vi "FormatTest.vi"(8 "entrée d'erreur (pas d'erreur)":errorcluster, 11 "read buffer en entrée":string) -> (0 "sortie d'erreur":errorcluster, 2 "result string":string)   [LabVIEW 2020]
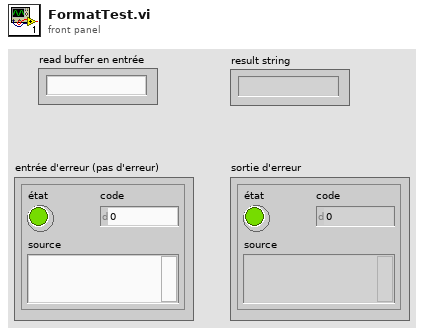
[diagram p1: front panel]
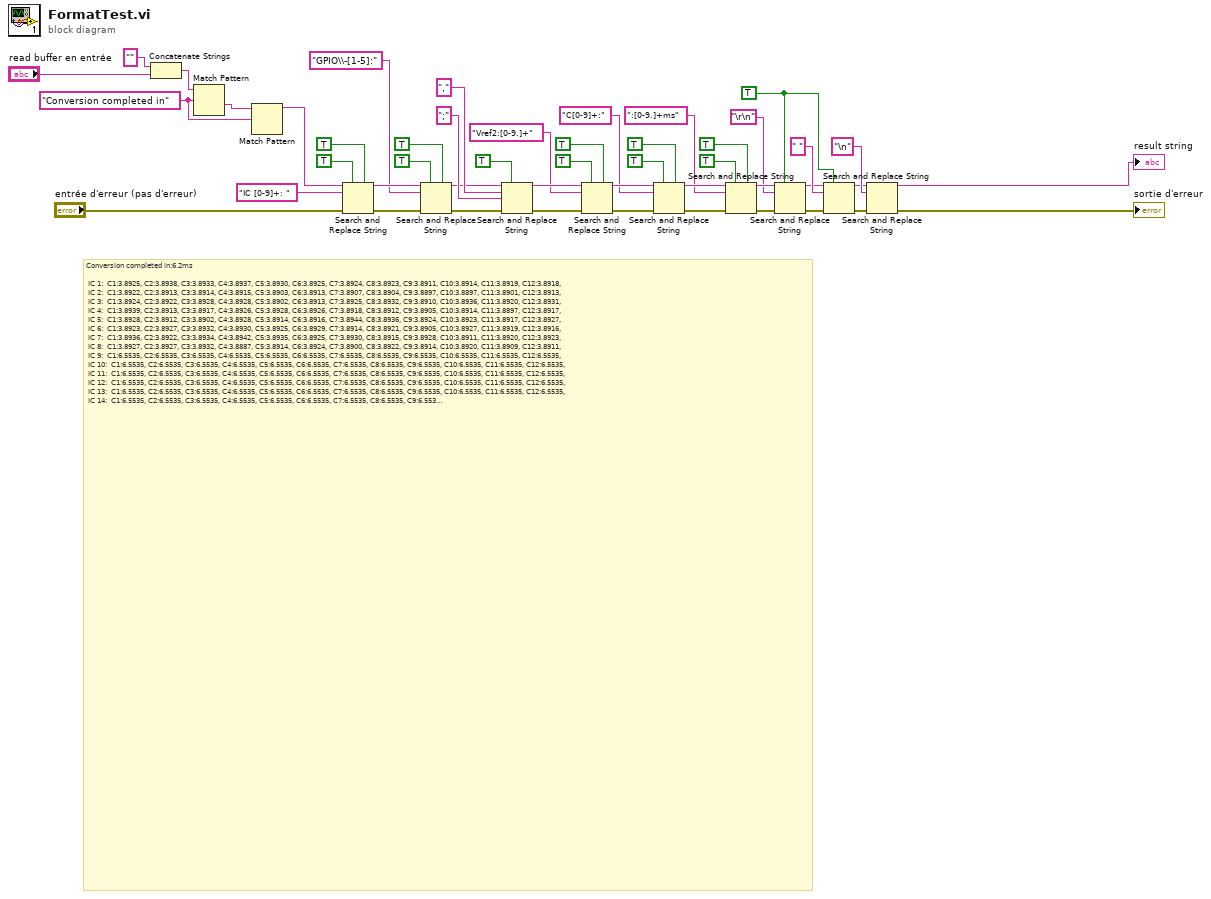
[diagram p0: block diagram]
diagram:
  w35 = "Conversion completed in" ("expression régulière")
  w24 = TRUE ("tout remplacer ? (F)")
  # "Conversion completed in:6.2ms \n\n IC 1:  C1:3.8925, C2:3.8938, C3:3.8933, C4:3.8937, C5:3.8930, C6:3.8925, C7:3.8924, C8:3.8923, C9:3.8911, C10:3.8914, C11:3.8919, C12:3.8918,\n IC 2:  C1:3.8922, C2:3.8913, C3:3.8914, C4:3.8915, C5:3.8903, C6:3.8913, C7:3.8907, C8:3.8904, C9:3.8897, C10:3.8897, C11:3.8901, C12:3.8913,\n IC 3:  C1:3.8924, C2:3.8922, C3:3.8928, C4:3.8928, C5:3.8902, C6:3.8913, C7:3.8925, C8:3.8932, C9:3.8910, C10:3.8936, C11:3.8920, C12:3.8931,\n IC 4:  C1:3.8939, C2:3.8913, C3:3.8917, C4:3.8926, C5:3.8928, C6:3.8926, C7:3.8918, C8:3.8912, C9:3.8905, C10:3.8914, C11:3.8897, C12:3.8917,\n IC 5:  C1:3.8928, C2:3.8912, C3:3.8902, C4:3.8928, C5:3.8914, C6:3.8916, C7:3.8944, C8:3.8936, C9:3.8924, C10:3.8923, C11:3.8917, C12:3.8927,\n IC 6:  C1:3.8923, C2:3.8927, C3:3.8932, C4:3.8930, C5:3.8925, C6:3.8929, C7:3.8914, C8:3.8921, C9:3.8905, C10:3.8927, C11:3.8919, C12:3.8916,\n IC 7:  C1:3.8936, C2:3.8922, C3:3.8934, C4:3.8942, C5:3.8935, C6:3.8925, C7:3.8930, C8:3.8915, C9:3.8928, C10:3.8911, C11:3.8920, C12:3.8923,\n IC 8:  C1:3.8927, C2:3.8927, C3:3.8932, C4:3.8887, C5:3.8914, C6:3.8924, C7:3.8900, C8:3.8922, C9:3.8914, C10:3.8920, C11:3.8909, C12:3.8911,\n IC 9:  C1:6.5535, C2:6.5535, C3:6.5535, C4:6.5535, C5:6.5535, C6:6.5535, C7:6.5535, C8:6.5535, C9:6.5535, C10:6.5535, C11:6.5535, C12:6.5535,\n IC 10:  C1:6.5535, C2:6.5535, C3:6.5535, C4:6.5535, C5:6.5535, C6:6.5535, C7:6.5535, C8:6.5535, C9:6.5535, C10:6.5535, C11:6.5535, C12:6.5535,\n IC 11:  C1:6.5535, C2:6.5535, C3:6.5535, C4:6.5535, C5:6.5535, C6:6.5535, C7:6.5535, C8:6.5535, C9:6.5535, C10:6.5535, C11:6.5535, C12:6.5535,\n IC 12:  C1:6.5535, C2:6.5535, C3:6.5535, C4:6.5535, C5:6.5535, C6:6.5535, C7:6.5535, C8:6.5535, C9:6.5535, C10:6.5535, C11:6.5535, C12:6.5535,\n IC 13:  C1:6.5535, C2:6.5535, C3:6.5535, C4:6.5535, C5:6.5535, C6:6.5535, C7:6.5535, C8:6.5535, C9:6.5535, C10:6.5535, C11:6.5535, C12:6.5535,\n IC 14:  C1:6.5535, C2:6.5535, C3:6.5535, C4:6.5535, C5:6.5535, C6:6.5535, C7:6.5535, C8:6.5535, C9:6.5535, C10:6.5535, C11:6.5535, C12:6.5535,\n IC 15:  C1:6.5535, C2:6.5535, C3:6.5535, C4:6.5535, C5:6.5535, C6:6.5535, C7:6.5535, C8:6.5535, C9:6.5535, C10:6.5535, C11:6.5535, C12:6.5535,\n IC 16:  C1:6.5535, C2:6.5535, C3:6.5535, C4:6.5535, C5:6.5535, C6:6.5535, C7:6.5535, C8:6.5535, C9:6.5535, C10:6.5535, C11:6.5535, C12:6.5535,\n IC 17:  C1:6.5535, C2:6.5535, C3:6.5535, C4:6.5535, C5:6.5535, C6:6.5535, C7:6.5535, C8:6.5535, C9:6.5535, C10:6.5535, C11:6.5535, C12:6.5535,\n IC 18:  C1:6.5535, C2:6.5535, C3:6.5535, C4:6.5535, C5:6.5535, C6:6.5535, C7:6.5535, C8:6.5535, C9:6.5535, C10:6.5535, C11:6.5535, C12:6.5535,\n\n\nConversion completed in:6.0ms \n\n IC 1: GPIO-1:1.2690, GPIO-2:1.7245, GPIO-3:1.2787, GPIO-4:1.7337, GPIO-5:2.9146, Vref2:3.0026\n IC 2: GPIO-1:1.2757, GPIO-2:1.7334, GPIO-3:1.2782, GPIO-4:1.7280, GPIO-5:2.9131, Vref2:3.0026\n IC 3: GPIO-1:1.2693, GPIO-2:1.7273, GPIO-3:1.2789, GPIO-4:1.7301, GPIO-5:2.9155, Vref2:3.0032\n IC 4: GPIO-1:1.2732, GPIO-2:1.7270, GPIO-3:1.2744, GPIO-4:1.7272, GPIO-5:2.9149, Vref2:3.0045\n IC 5: GPIO-1:1.2722, GPIO-2:1.7276, GPIO-3:1.2787, GPIO-4:1.7338, GPIO-5:2.9154, Vref2:3.0037\n IC 6: GPIO-1:1.2798, GPIO-2:1.7296, GPIO-3:1.2777, GPIO-4:1.7339, GPIO-5:2.9154, Vref2:3.0022\n IC 7: GPIO-1:1.2744, GPIO-2:1.7332, GPIO-3:1.2821, GPIO-4:1.7290, GPIO-5:2.9165, Vref2:3.0042\n IC 8: GPIO-1:1.2800, GPIO-2:1.7290, GPIO-3:1.2835, GPIO-4:1.7244, GPIO-5:2.9148, Vref2:3.0027\n IC 9: GPIO-1:6.5535, GPIO-2:6.5535, GPIO-3:6.5535, GPIO-4:6.5535, GPIO-5:6.5535, Vref2:6.5535\n IC 10: GPIO-1:6.5535, GPIO-2:6.5535, GPIO-3:6.5535, GPIO-4:6.5535, GPIO-5:6.5535, Vref2:6.5535\n IC 11: GPIO-1:6.5535, GPIO-2:6.5535, GPIO-3:6.5535, GPIO-4:6.5535, GPIO-5:6.5535, Vref2:6.5535\n IC 12: GPIO-1:6.5535, GPIO-2:6.5535, GPIO-3:6.5535, GPIO-4:6.5535, GPIO-5:6.5535, Vref2:6.5535\n IC 13: GPIO-1:6.5535, GPIO-2:6.5535, GPIO-3:6.5535, GPIO-4:6.5535, GPIO-5:6.5535, Vref2:6.5535\n IC 14: GPIO-1:6.5535, GPIO-2:6.5535, GPIO-3:6.5535, GPIO-4:6.5535, GPIO-5:6.5535, Vref2:6.5535\n IC 15: GPIO-1:6.5535, GPIO-2:6.5535, GPIO-3:6.5535, GPIO-4:6.5535, GPIO-5:6.5535, Vref2:6.5535\n IC 16: GPIO-1:6.5535, GPIO-2:6.5535, GPIO-3:6.5535, GPIO-4:6.5535, GPIO-5:6.5535, Vref2:6.5535\n IC 17: GPIO-1:6.5535, GPIO-2:6.5535, GPIO-3:6.5535, GPIO-4:6.5535, GPIO-5:6.5535, Vref2:6.5535\n IC 18: GPIO-1:6.5535, GPIO-2:6.5535, GPIO-3:6.5535, GPIO-4:6.5535, GPIO-5:6.5535, Vref2:6.5535"
  n1 = Concatenate Strings("", "read buffer en entrée") -> (w36:string)
  n2 = Match Pattern ("Rechercher une expression")(string=w36, regular expression=w35) -> (after substring=w34:string)  [unwired: 1 in, 3 out]
  n3 = Match Pattern ("Rechercher une expression")(string=w34, regular expression=w35) -> (before substring=w46:string)  [unwired: 1 in, 3 out]
  n4 = Search and Replace String ("Rechercher et remplacer une chaîne")(replace all?=TRUE ("tout remplacer ? (F)"), multiline?=TRUE ("multiligne ? (F)"), input string=w46, search string="IC [0-9]+: " ("chaîne recherchée"), error in="entrée d'erreur (pas d'erreur)") -> (result string=w8:string, error out=w37:errorcluster)  [unwired: 3 in, 2 out]
  n5 = Search and Replace String ("Rechercher et remplacer une chaîne")(replace all?=TRUE ("tout remplacer ? (F)"), multiline?=TRUE ("multiligne ? (F)"), input string=w8, search string="GPIO\\-[1-5]:" ("chaîne recherchée"), error in=w37) -> (result string=w28:string, error out=w38:errorcluster)  [unwired: 3 in, 2 out]
  n6 = Search and Replace String ("Rechercher et remplacer une chaîne")(replace all?=TRUE ("tout remplacer ? (F)"), input string=w28, search string="," ("chaîne recherchée"), replace string=";" ("chaîne de remplacement (\"\")"), error in=w38) -> (result string=w29:string, error out=w39:errorcluster)  [unwired: 3 in, 2 out]
  n7 = Search and Replace String ("Rechercher et remplacer une chaîne")(replace all?=TRUE ("tout remplacer ? (F)"), multiline?=TRUE ("multiligne ? (F)"), input string=w29, search string="Vref2:[0-9.]+" ("chaîne recherchée"), error in=w39) -> (result string=w15:string, error out=w40:errorcluster)  [unwired: 3 in, 2 out]
  n8 = Search and Replace String ("Rechercher et remplacer une chaîne")(replace all?=TRUE ("tout remplacer ? (F)"), multiline?=TRUE ("multiligne ? (F)"), input string=w15, search string="C[0-9]+:" ("chaîne recherchée"), error in=w40) -> (result string=w17:string, error out=w41:errorcluster)  [unwired: 3 in, 2 out]
  n9 = Search and Replace String ("Rechercher et remplacer une chaîne")(replace all?=TRUE ("tout remplacer ? (F)"), multiline?=TRUE ("multiligne ? (F)"), input string=w17, search string=":[0-9.]+ms" ("chaîne recherchée"), error in=w41) -> (result string=w21:string, error out=w42:errorcluster)  [unwired: 3 in, 2 out]
  n10 = Search and Replace String ("Rechercher et remplacer une chaîne")(replace all?=w24, input string=w21, search string="\r\n", error in=w42) -> (result string=w22:string, error out=w44:errorcluster)  [unwired: 4 in, 2 out]
  n11 = Search and Replace String ("Rechercher et remplacer une chaîne")(replace all?=w24, input string=w22, search string=" " ("chaîne recherchée"), error in=w44) -> (result string=w25:string, error out=w43:errorcluster)  [unwired: 4 in, 2 out]
  n12 = Search and Replace String ("Rechercher et remplacer une chaîne")(input string=w25, search string="\n" ("chaîne recherchée"), error in=w43) -> (result string=→"result string":string, error out=→"sortie d'erreur":errorcluster)  [unwired: 5 in, 2 out]
